vi "InitAxisPanels(SubVI).vi"(8 "error in (no error)":errorcluster) -> (0 "error out":errorcluster, 3 "AxisControlSubPanelRef":refnum<vi>)   [LabVIEW 2020]
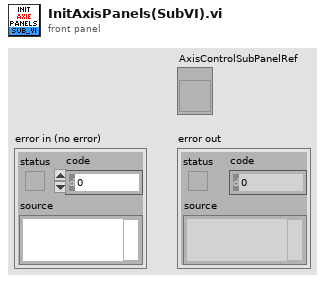
[diagram p1: front panel]
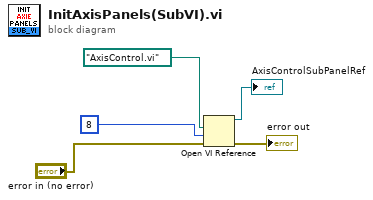
[diagram p0: block diagram]
diagram:
  n1 = Open VI Reference(vi path=path "AxisControl.vi", options=8, error in (no error)="error in (no error)") -> (vi reference=→"AxisControlSubPanelRef":refnum<vi>, error out=→"error out":errorcluster)  [unwired: 3 in]
